vi "tm420_sequence_wVision.vi"() -> ()   [LabVIEW 2011]
panel:
  out "Display":T1(plugin-control)
  out "Timestamp":dbl
  out "DCAM Version":string
  out "Library Version":string
  out "Frames Per Second":dbl
  in  "Quit":bool
  out "Error Out":errorcluster {"code" format="%.0x"}
  # "This is just a simple example\nof how to capture and display\nlive data."
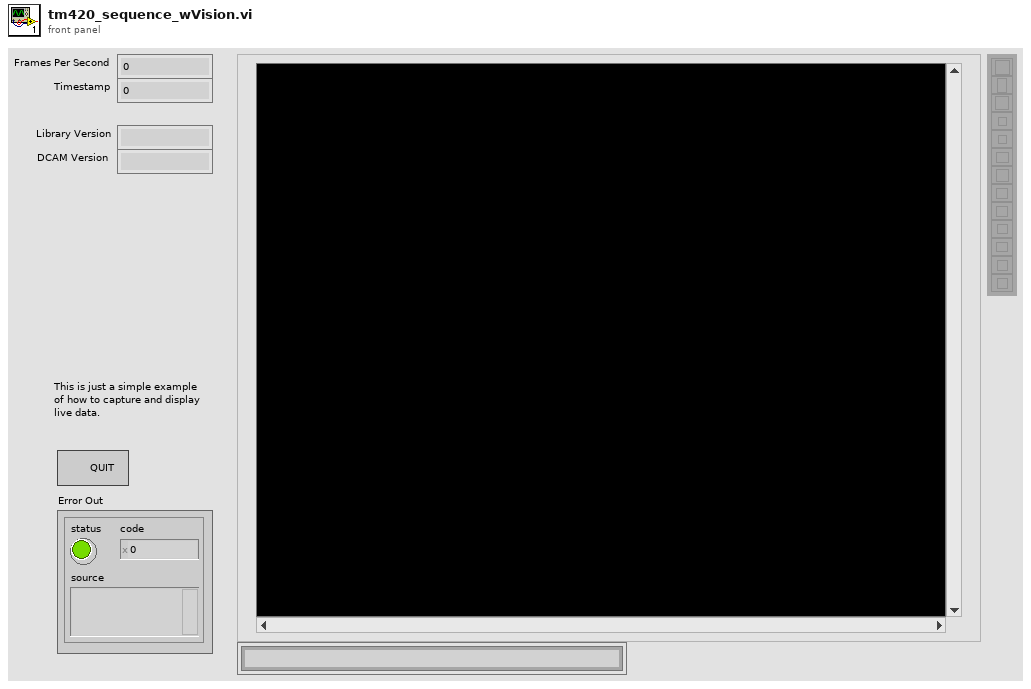
[diagram p1: front panel]
types:
  T1 = typedef "IMAQ Image.ctl" = refnum<image>
  T2 = cluster{"Capture Library":string, "DCAM-API":string}
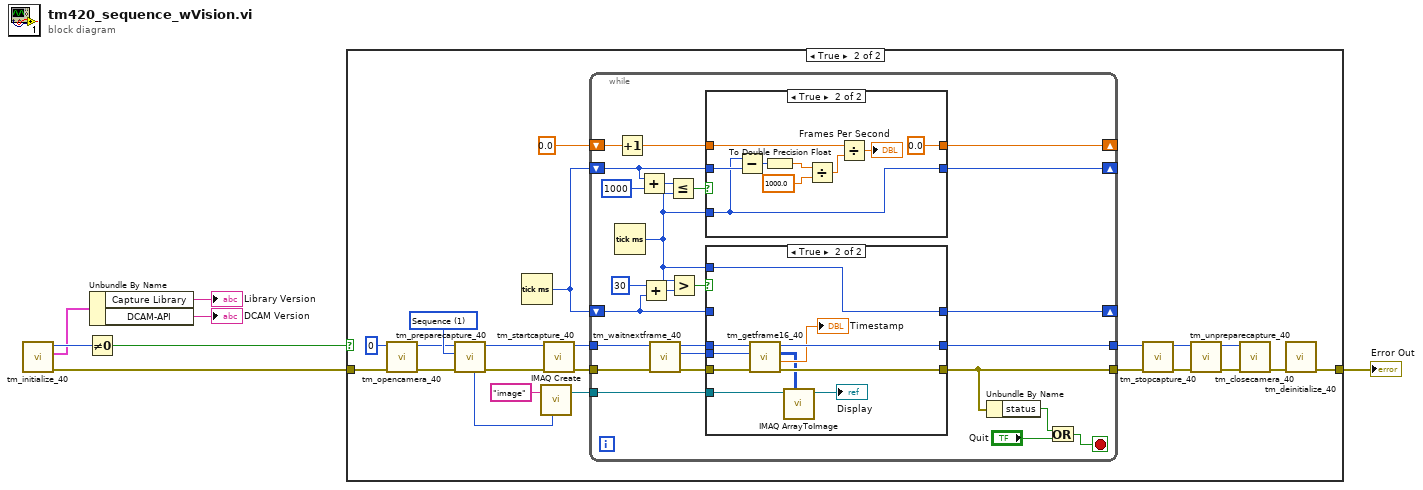
[diagram p0: block diagram]
diagram:
  n1 = call <userlib>:"tm_initialize_40.vi"() -> ("error out"=w4:errorcluster, "Version Info"=w3:T2, "Number Of Cameras"=w5:u32)  [unwired: 8 in, 1 out]
  n2 = Not Equal To 0?(x=w5) -> (x != 0?=w7:bool)
  n3 = Unbundle By Name(w3) -> ("Capture Library"=→"Library Version":string, "DCAM-API"=→"DCAM Version":string)
  n4 = case shown="True" w7 {
    tunnel: w4 -> [w8 w30]
    tunnel: [w8 w27] -> w6
    frame False {
    }
    frame True {
      w18 = 1 items=["Snap", "Sequence"] ("Capture mode")
      n5 = call <userlib>:"tm_opencamera_40.vi"("error in (no error)"=w30, "Camera Index"=u32 0) -> ("error out"=w12:errorcluster, "Handle out"=w13:u32)  [unwired: 7 in, 1 out]
      n6 = call <userlib>:"tm_preparecapture_40.vi"("error in (no error)"=w12, "Capture mode"=w18, "Handle in"=w13) -> ("error out"=w16:errorcluster, "Handle out"=w17:u32, "Image type"=w10:u32)  [unwired: 5 in, 1 out]
      n7 = Tick Count (ms)() -> (millisecond timer value=w14:u32)
      n8 = call "IMAQ Create"("Image Name"="image", "Image Type"=w10) -> ("New Image"=w9:T1)  [unwired: 3 in, 1 out]
      n9 = call <userlib>:"tm_startcapture_40.vi"("error in (no error)"=w16, "Handle in"=w17) -> ("error out"=w19:errorcluster, "Handle out"=w20:u32)  [unwired: 8 in]
      n10 = while {
        tunnel: [w34] -> w23
        tunnel: [w35] -> w24
        tunnel: w20 -> [w52]
        tunnel: w19 -> [w53]
        shift-right: [w50] -> _
        shift-left: w14 -> [w47]
        shift-right: [w51] -> _
        shift-left: 0.0 -> [w44]
        shift-right: [w33] -> _
        shift-left: w14 -> [w36]
        tunnel: w9 -> [w32]
        stop <- w31 stop-if-true
        n11 = Tick Count (ms)() -> (millisecond timer value=w37:u32)
        n12 = Increment(x=w44) -> (x+1=w45:dbl)
        n13 = Add(x=w47, y=u32 1000) -> (x+y=w49:u32)
        n14 = Add(x=u32 30, y=w36) -> (x+y=w39:u32)
        n15 = call <userlib>:"tm_waitnextframe_40.vi"("error in (no error)"=w53, "Handle in"=w52) -> ("error out"=w42:errorcluster, "Frame Index"=w41:i32, "Handle out"=w43:u32)  [unwired: 6 in, 1 out]
        n16 = Less Or Equal?(x=w49, y=w37) -> (x <= y?=w46:bool)
        n17 = Greater?(x=w37, y=w39) -> (0:w38:bool)
        n18 = case shown="True" w46 {
          tunnel: w47 -> [w70 w73]
          tunnel: [w70 w71] -> w50
          tunnel: w45 -> [w69 w77]
          tunnel: w37 -> [_ w71]
          tunnel: [w69 0.0] -> w51
          frame False {
          }
          frame True {
            n19 = Subtract(x=w71, y=w73) -> (x-y=w72:u32)
            n20 = To Double Precision Float(number=w72) -> (double precision float=w79:dbl)
            n21 = Divide(x=w79, y=1000.0) -> (x/y=w76:dbl)
            n22 = Divide(x=w77, y=w76) -> (x/y=→"Frames Per Second":dbl)
          }
        }
        n23 = case shown="True" w38 {
          tunnel: w43 -> [w58 w68]
          tunnel: w42 -> [w57 w67]
          tunnel: w41 -> [_ w62]
          tunnel: w36 -> [w56 _]
          tunnel: w37 -> [_ w66]
          tunnel: [w58 w64] -> w34
          tunnel: [w57 w65] -> w35
          tunnel: [w56 w66] -> w33
          tunnel: w32 -> [_ w61]
          frame False {
          }
          frame True {
            n24 = call <userlib>:"tm_getframe16_40.vi"("error in (no error)"=w67, "Frame Index"=w62, "Handle in"=w68) -> ("error out"=w65:errorcluster, "Timestamp"=→"Timestamp":dbl, "Data"=w60:u16[][], "Handle out"=w64:u32)  [unwired: 5 in]
            n25 = call "IMAQ ArrayToImage"("Image Pixels (U16)"=w60, "Image"=w61) -> ("Image Out"=→"Display":T1)  [unwired: 8 in, 1 out]
          }
        }
        n26 = Unbundle By Name(w35) -> ("status"=w55:bool)
        n27 = Or(x=w55, y="Quit") -> (x .or. y?=w31:bool)
      }
      n28 = call <userlib>:"tm_stopcapture_40.vi"("error in (no error)"=w24, "Handle in"=w23) -> ("error out"=w21:errorcluster, "Handle out"=w22:u32)  [unwired: 8 in]
      n29 = call <userlib>:"tm_unpreparecapture_40.vi"("error in (no error)"=w21, "Handle in"=w22) -> ("error out"=w26:errorcluster, "Handle out"=w25:u32)  [unwired: 8 in]
      n30 = call <userlib>:"tm_closecamera_40.vi"("error in (no error)"=w26, "Handle in"=w25) -> ("error out"=w28:errorcluster)  [unwired: 9 in]
      n31 = call <userlib>:"tm_deinitialize_40.vi"("error in (no error)"=w28) -> ("error out"=w27:errorcluster)  [unwired: 10 in]
    }
  }
  "Error Out" <- w6
